vi "dfd_Lp Norm Params Validation.vi"(4 "max pole radius":dbl=0.95 min=0.0, 6 "fs [Hz]":dbl=1.0 format="%.2f", 8 "error in (no error)":errorcluster, 9 "p":i32=128, 10 "bands spec":T1 {"magnitude and weight"."frequency point"."weight" format="%.2f"}, 11 "order":cluster{"num":i32, "den":i32}={"num"=5, "den"=5}) -> (0 "error out":errorcluster, 1 "p out":i32=128, 2 "dup bands spec":T1 {"magnitude and weight"."frequency point"."weight" format="%.2f"}, 3 "dup order":cluster{"num":i32, "den":i32}={"num"=5, "den"=5})   [LabVIEW 2017, in "NI_DigFilterLicensed.lvlib"]
uses:
  <vilib>/addons/Digital Filter Design/NI_DigFilterLicensed.lvlib
  <vilib>/addons/Digital Filter Design/_LpNorm.llb/dfd_Lp Norm Band Spec.ctl
  <vilib>/addons/Digital Filter Design/_Misc.llb/dfd_Error Handlers (Multiple).vi
panel:
  # "frequency"
  # "magnitude"
  # "weight"
  # "phase"
  # "frequency"
  # "magnitude"
  # "weight"
  # "phase"
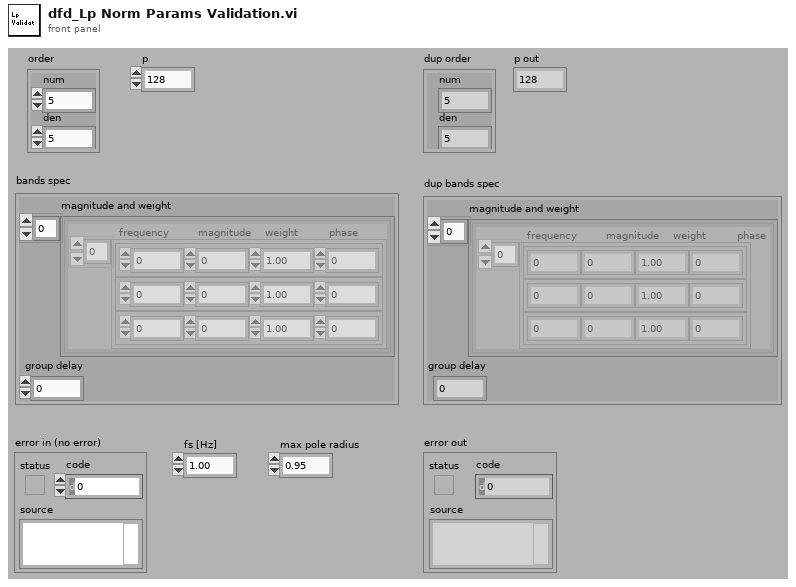
[diagram p1: front panel]
types:
  T1 = typedef "dfd_Lp Norm Band Spec.ctl" = cluster{"magnitude and weight":cluster{"frequency point":cluster{"frequency":dbl, "magnitude":dbl, "weight":dbl, "phase":dbl}[]}[], "group delay":dbl}
  T2 = cluster{"frequency point":cluster{"frequency":dbl, "magnitude":dbl, "weight":dbl, "phase":dbl}[]}[]
  T3 = cluster{"frequency":dbl, "magnitude":dbl, "weight":dbl, "phase":dbl}[]
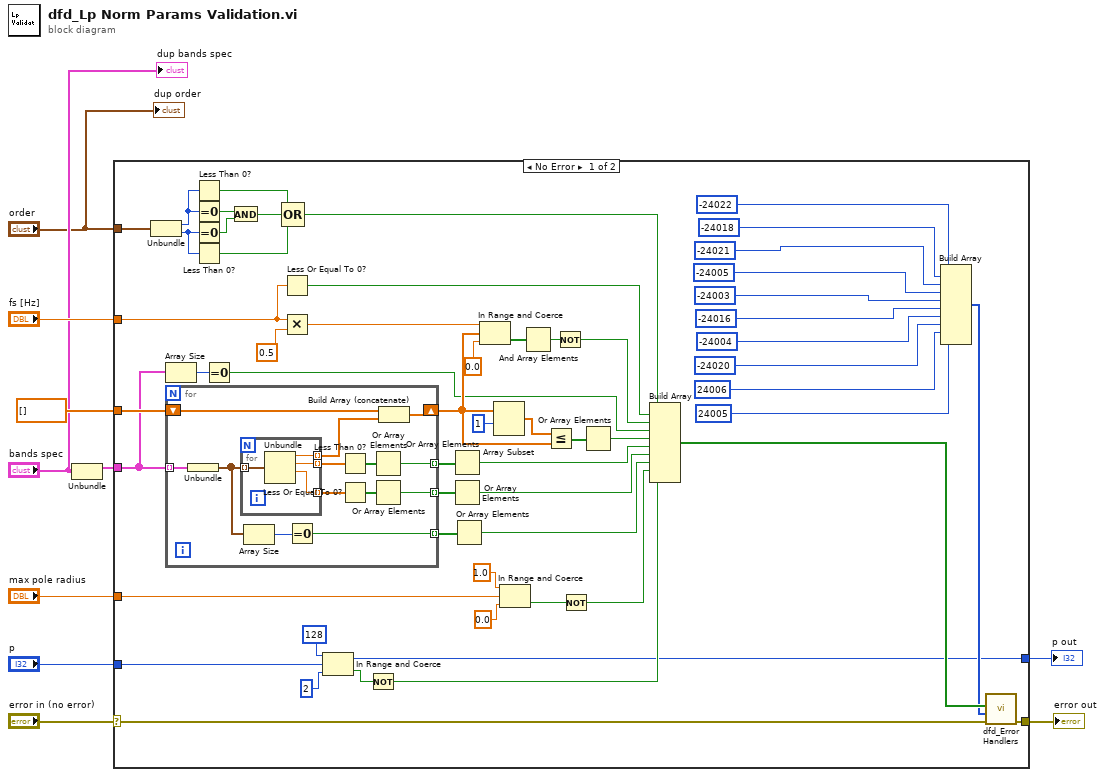
[diagram p0: block diagram]
diagram:
  n1 = Unbundle("bands spec") -> ("magnitude and weight"=w1:T2)  [unwired: 1 out]
  n2 = case shown="No Error" "error in (no error)" {
    selector: "error in (no error)" -> [w32 w85]
    tunnel: dbl[] [] -> [w67 _]
    tunnel: "fs [Hz]" -> [w52 _]
    tunnel: [w49 w85] -> w8
    tunnel: "p" -> [w17 w86]
    tunnel: [w16 w86] -> w6
    tunnel: w1 -> [w15 _]
    tunnel: "order" -> [w37 _]
    tunnel: "max pole radius" -> [w36 _]
    frame No Error {
      n3 = Unbundle(w37) -> ("num"=w44:i32, "den"=w45:i32)
      n4 = Array Size(array=w15) -> (size(s)=w14:i32)
      n5 = for {
        tunnel: w15 -> [w80] mode=indexing
        shift-right: [w77] -> w59
        shift-left: w67 -> [w79]
        tunnel: [w72] -> w63 mode=indexing
        tunnel: [w71] -> w62 mode=indexing
        tunnel: [w68] -> w22 mode=indexing
        n6 = Unbundle(w80) -> ("frequency point"=w70:T3)
        n7 = for {
          tunnel: w70 -> [w84] mode=indexing
          tunnel: [w83] -> w78 mode=indexing
          tunnel: [w82] -> w76 mode=indexing
          tunnel: [w81] -> w75 mode=indexing
          n8 = Unbundle(w84) -> ("frequency"=w83:dbl, "magnitude"=w82:dbl, "weight"=w81:dbl)  [unwired: 1 out]
        }
        n9 = Array Size(array=w70) -> (size(s)=w69:i32)
        n10 = Equal To 0?(x=w69) -> (x = 0?=w68:bool)
        n11 = Less Than 0?(x=w76) -> (x < 0?=w74:bool[])
        n12 = Less Or Equal To 0?(x=w75) -> (x <= 0?=w73:bool[])
        n13 = Or Array Elements(Boolean array=w74) -> (logical OR=w72:bool)
        n14 = Or Array Elements(Boolean array=w73) -> (logical OR=w71:bool)
        n15 = Build Array (concatenate)(w79, w78) -> (w77:dbl[])
      }
      n16 = Less Than 0?(x=w44) -> (x < 0?=w41:bool)
      n17 = Equal To 0?(x=w44) -> (x = 0?=w43:bool)
      n18 = Equal To 0?(x=w45) -> (x = 0?=w42:bool)
      n19 = Less Than 0?(x=w45) -> (x < 0?=w39:bool)
      n20 = Equal To 0?(x=w14) -> (x = 0?=w12:bool)
      n21 = And(x=w43, y=w42) -> (x .and. y?=w40:bool)
      n22 = Compound Arithmetic op=OR(w41, w40, w39) -> (w38:bool)
      n23 = Less Or Equal To 0?(x=w52) -> (x <= 0?=w50:bool)
      n24 = Multiply(x=w52, y=0.5) -> (x*y=w54:dbl)
      n25 = In Range and Coerce(upper limit=128, x=w17, lower limit=2) -> (coerced(x)=w16:i32, In Range?=w46:bool)
      n26 = Not(x=w46) -> (.not. x?=w33:bool)
      n27 = Or Array Elements(Boolean array=w63) -> (logical OR=w57:bool)
      n28 = Or Array Elements(Boolean array=w62) -> (logical OR=w56:bool)
      n29 = Or Array Elements(Boolean array=w22) -> (logical OR=w21:bool)
      n30 = In Range and Coerce(upper limit=w54, x=w59, lower limit=0.0) -> (In Range?=w65:bool[])  [unwired: 1 out]
      n31 = Array Subset(array=w59, index=1) -> (w60:dbl[])  [unwired: 1 in]
      n32 = In Range and Coerce(upper limit=1.0, x=w36, lower limit=0.0) -> (In Range?=w19:bool)  [unwired: 1 out]
      n33 = And Array Elements(Boolean array=w65) -> (logical AND=w64:bool)
      n34 = Less Or Equal?(x=w60, y=w59) -> (x <= y?=w58:bool[])
      n35 = Not(x=w64) -> (.not. x?=w51:bool)
      n36 = Not(x=w19) -> (.not. x?=w34:bool)
      n37 = Or Array Elements(Boolean array=w58) -> (logical OR=w13:bool)
      n38 = Build Array(w38, w50, w51, w12, w13, w57, w56, w21, w34, w33) -> (w55:bool[])
      n39 = Build Array(-24022 ("ERR_ORDER_LE_ZERO"), -24018 ("ERR_FS_LE_ZERO"), -24021 ("ERR_FREQ_RANGE_WRONG"), -24005 ("ERR_EMPTY_BAND"), -24003 ("ERR_BAND_FREQ_SEG_WRONG"), -24016 ("ERR_MAG_LT_ZERO"), -24004 ("ERR_WEIGHT_LE_ZERO"), -24020 ("ERR_INVALID_BAND"), 24006 ("WRN_RAIUS_RANGE"), 24005 ("WRN_P_RANGE")) -> (w23:i32[])
      n40 = call-poly <vilib>:"dfd_Error Handlers.vi"("error in (no error)"=w32, "error sources"=w23, "condition failed?"=w55) -> ("error out"=w49:errorcluster)  [unwired: 8 out]
    }
    frame Error {
    }
  }
  "error out" <- w8
  "p out" <- w6
  "dup bands spec" <- "bands spec"
  "dup order" <- "order"
